vi "Register gRPC Methods.vi"(8 "error in (no error)":errorcluster, 11 "gRPC service in":refnum<class "ExamplePluginOOBService.lvclass">) -> (0 "error out":errorcluster, 3 "gRPC service out":refnum<class "ExamplePluginOOBService.lvclass">)   [LabVIEW 2025, in "Automotive-Vision-OOBService_server.lvlib" / "ExamplePluginOOBService.lvclass"]
uses:
  ExamplePluginOOBService.lvclass
  typeDefs/Server Internal UEs.ctl
  typeDefs/Server Internal Message.ctl
  typeDefs/Server gRPC UEs.ctl
  <vilib>/gRPC/LabVIEW gRPC Library/Server API/typeDefs/gRPCId Cluster.ctl
  <vilib>/gRPC/LabVIEW gRPC Library/Shared/grpcId.ctl
  ExamplePluginOOBService.lvclass/ExamplePluginOOBService.ctl
  <vilib>/gRPC/LabVIEW gRPC Library/grpc-lvsupport-release.lvlib
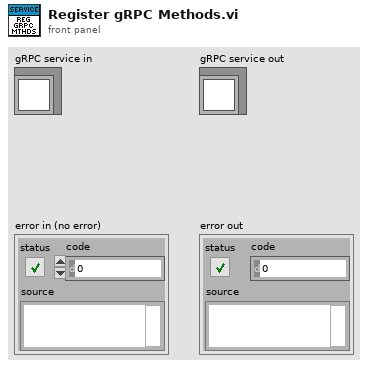
[diagram p1: front panel]
types:
  T1 = typedef "Automotive-Vision-OOBService_server.lvlib/ExamplePluginOOBService.lvclass/Server gRPC UEs.ctl" = cluster{"ExamplePluginOOBService PauseResume gRPC UE":refnum<user-event>, "ExamplePluginOOBService ExportPath gRPC UE":refnum<user-event>, "ExamplePluginOOBService ExportType gRPC UE":refnum<user-event>, "ExamplePluginOOBService Export gRPC UE":refnum<user-event>}
  T2 = typedef "Automotive-Vision-OOBService_server.lvlib/ExamplePluginOOBService.lvclass/Server Internal UEs.ctl" = cluster{"ExamplePluginOOBService PauseResume Internal UE":refnum<user-event>, "ExamplePluginOOBService ExportPath Internal UE":refnum<user-event>, "ExamplePluginOOBService ExportType Internal UE":refnum<user-event>, "ExamplePluginOOBService Export Internal UE":refnum<user-event>}
  T3 = typedef "grpc-lvsupport-release.lvlib/grpcId.ctl" = u64
  T4 = typedef "Automotive-Vision-OOBService_server.lvlib/ExamplePluginOOBService.lvclass/Server Internal Message UE.ctl" = refnum<user-event>
  T5 = typedef "grpc-lvsupport-release.lvlib/gRPCId Cluster UE.ctl" = refnum<user-event>
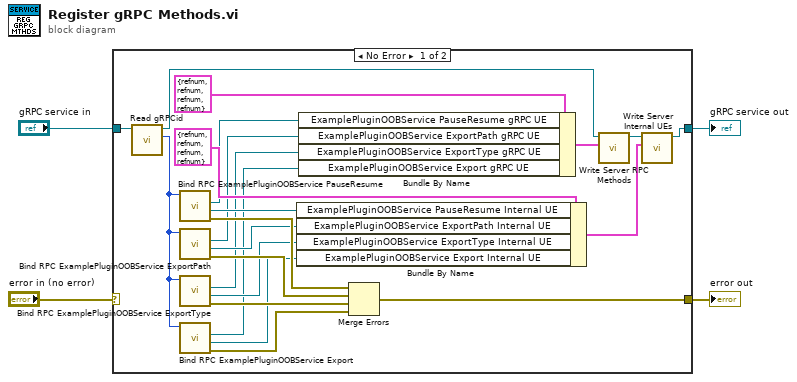
[diagram p0: block diagram]
diagram:
  n1 = case shown="No Error" "error in (no error)" {
    selector: "error in (no error)" -> [_ w27]
    tunnel: "gRPC service in" -> [w18 w28]
    tunnel: [w26 w27] -> w3
    tunnel: [w25 w28] -> w2
    frame No Error {
      n2 = call-dynamic "Read gRPCid.vi"("gRPC service in"=w18) -> ("gRPCid"=w17:T3, "gRPC service out"=w19:refnum<class "ExamplePluginOOBService.lvclass">)  [unwired: 8 in, 1 out]
      n3 = call "Bind RPC ExamplePluginOOBService PauseResume.vi"("gRPCid server in"=w17) -> ("error out"=w16:errorcluster, "ExamplePluginOOBService PauseResume Internal UE"=w14:T4, "ExamplePluginOOBService PauseResume gRPC UE"=w15:T5)  [unwired: 7 in, 1 out]
      n4 = call "Bind RPC ExamplePluginOOBService ExportPath.vi"("gRPCid server in"=w17) -> ("error out"=w13:errorcluster, "ExamplePluginOOBService ExportPath Internal UE"=w11:T4, "ExamplePluginOOBService ExportPath gRPC UE"=w12:T5)  [unwired: 7 in, 1 out]
      n5 = call "Bind RPC ExamplePluginOOBService ExportType.vi"("gRPCid server in"=w17) -> ("error out"=w10:errorcluster, "ExamplePluginOOBService ExportType Internal UE"=w8:T4, "ExamplePluginOOBService ExportType gRPC UE"=w9:T5)  [unwired: 7 in, 1 out]
      n6 = call "Bind RPC ExamplePluginOOBService Export.vi"("gRPCid server in"=w17) -> ("error out"=w7:errorcluster, "ExamplePluginOOBService Export Internal UE"=w5:T4, "ExamplePluginOOBService Export gRPC UE"=w6:T5)  [unwired: 7 in, 1 out]
      n7 = Bundle By Name ("Bundle Internal UEs")(cluster=T2 {"ExamplePluginOOBService PauseResume Internal UE"=refnum, "ExamplePluginOOBService ExportPath Internal UE"=refnum, "ExamplePluginOOBService ExportType Internal UE"=refnum, "ExamplePluginOOBService Export Internal UE"=refnum} ("Server Internal UEs"), "ExamplePluginOOBService PauseResume Internal UE"=w14, "ExamplePluginOOBService ExportPath Internal UE"=w11, "ExamplePluginOOBService ExportType Internal UE"=w8, "ExamplePluginOOBService Export Internal UE"=w5) -> (w24:T2)
      n8 = Bundle By Name ("Bundle gRPC UEs")(cluster=T1 {"ExamplePluginOOBService PauseResume gRPC UE"=refnum, "ExamplePluginOOBService ExportPath gRPC UE"=refnum, "ExamplePluginOOBService ExportType gRPC UE"=refnum, "ExamplePluginOOBService Export gRPC UE"=refnum} ("gRPC Server Method Events"), "ExamplePluginOOBService PauseResume gRPC UE"=w15, "ExamplePluginOOBService ExportPath gRPC UE"=w12, "ExamplePluginOOBService ExportType gRPC UE"=w9, "ExamplePluginOOBService Export gRPC UE"=w6) -> (w21:T1)
      n9 = Merge Errors(w16, w13, w10, w7) -> (w26:errorcluster)
      n10 = call "Write Server RPC Methods.vi"("Server RPC Methods"=w21, "gRPC service in"=w19) -> ("gRPC service out"=w22:refnum<class "ExamplePluginOOBService.lvclass">)  [unwired: 8 in, 1 out]
      n11 = call "Write Server Internal UEs.vi"("Server Internal UEs"=w24, "gRPC service in"=w22) -> ("gRPC service out"=w25:refnum<class "ExamplePluginOOBService.lvclass">)  [unwired: 8 in, 1 out]
    }
    frame Error {
    }
  }
  "error out" <- w3
  "gRPC service out" <- w2
